vi "solar_excel Cell Escape.vi"(7 "Action (Escape)":enum8{"Escape", "Unescape"}(ring), 11 "String in":string) -> (3 "String out":string)   [LabVIEW 2018]
doc: "This escapes special Excel characters."
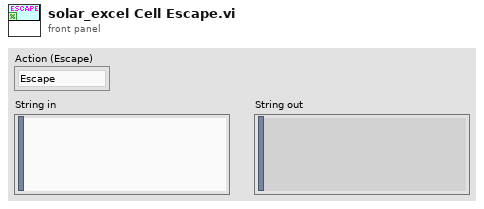
[diagram p1: front panel]
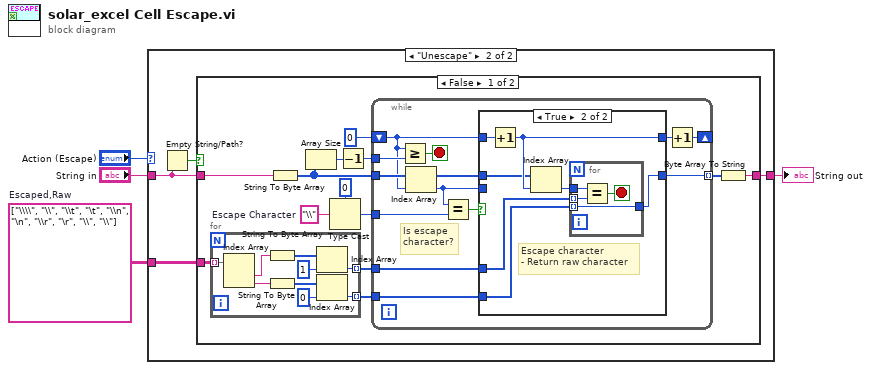
[diagram p0: block diagram]
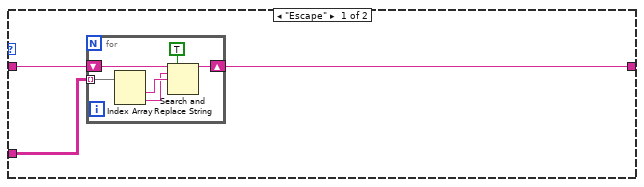
[diagram p2: hidden frame]
diagram:
  w1 = string[][] [["\\\\", "\\"], ["\\t", "\t"], ["\\n", "\n"], ["\\r", "\r"], ["\\", "\\"]]  # Escaped,Raw
  n1 = case shown="\"Unescape\"" "Action (Escape)" {
    tunnel: [w7 w17] -> w4
    tunnel: "String in" -> [w6 w15]
    tunnel: w1 -> [w5 w16]
    frame "Escape" {
      n2 = for {
        shift-right: [w11] -> w7
        shift-left: w6 -> [w12]
        tunnel: w5 -> [w10] mode=indexing
        n3 = Index Array(array=w10) -> (element #1=w9:string, element #2=w8:string)  [unwired: 2 in]
        n4 = Search and Replace String(replace all?=TRUE ("replace all? (F)"), input string=w12, search string=w8, replace string=w9) -> (result string=w11:string)  [unwired: 1 in, 6 out]
      }
    }
    frame "Unescape" {
      n5 = Empty String/Path?(string/path=w15) -> (empty?=w14:bool)
      n6 = case shown="False" w14 {
        tunnel: w15 -> [w30 w65]
        tunnel: [w21 w65] -> w17
        tunnel: w16 -> [w19 _]
        frame False {
          w29 = "\\"  # Escape Character
          n7 = for {
            tunnel: [w38] -> w20 mode=indexing
            tunnel: w19 -> [w36] mode=indexing
            tunnel: [w31] -> w18 mode=indexing
            n8 = Index Array(array=w36) -> (element #1=w32:string, element #2=w35:string)  [unwired: 2 in]
            n9 = String To Byte Array(string=w32) -> (unsigned byte array=w33:u8[])
            n10 = String To Byte Array(string=w35) -> (unsigned byte array=w39:u8[])
            n11 = Index Array(array=w33, index=1) -> (element=w31:u8)
            n12 = Index Array(array=w39, index=0) -> (element=w38:u8)
          }
          n13 = String To Byte Array(string=w30) -> (unsigned byte array=w23:u8[])
          n14 = Array Size(array=w23) -> (size(s)=w26:i32)
          n15 = Type Cast(type=u8 0, x=w29) -> (*(type *) &x=w22:u8)
          n16 = Decrement(x=w26) -> (x-1=w27:i32)
          n17 = while {
            shift-right: [w51] -> _
            shift-left: 0 ("index") -> [w46]
            tunnel: w23 -> [w49]
            tunnel: [w48] -> w24 mode=indexing
            tunnel: w27 -> [w47]
            tunnel: w22 -> [w44]
            tunnel: w18 -> [w41]
            tunnel: w20 -> [w40]
            stop <- w45 stop-if-true
            # "Is escape\ncharacter?"
            n18 = Greater Or Equal?(x=w46, y=w47) -> (x >= y?=w45:bool)
            n19 = Index Array(array=w49, index=w46) -> (element=w42:u8)
            n20 = Equal?(x=w42, y=w44) -> (x = y?=w43:bool)
            n21 = case shown="True" w43 {
              tunnel: w46 -> [w53 w60]
              tunnel: [w52 w54] -> w48
              tunnel: [w53 w59] -> w50
              tunnel: w49 -> [_ w58]
              tunnel: w42 -> [w52 _]
              tunnel: w41 -> [_ w57]
              tunnel: w40 -> [_ w55]
              frame False {
                # "Not escape character\n- Return original char"
              }
              frame True {
                # "Escape character\n- Return raw character"
                n22 = Increment(x=w60) -> (x+1=w59:i32)
                n23 = Index Array(array=w58, index=w59) -> (element=w56:u8)
                n24 = for {
                  tunnel: w57 -> [w63] mode=indexing
                  tunnel: w56 -> [w64]
                  tunnel: w55 -> [w62] mode=indexing
                  tunnel: [w62] -> w54
                  stop <- w61 stop-if-true
                  n25 = Equal?(x=w64, y=w63) -> (x = y?=w61:bool)
                }
              }
            }
            n26 = Increment(x=w50) -> (x+1=w51:i32)
          }
          n27 = Byte Array To String(unsigned byte array=w24) -> (string=w21:string)
        }
        frame True {
        }
      }
    }
  }
  "String out" <- w4
